vi "Close.vi"(8 "error in (no error)":errorcluster, 11 "PS Driver AMI4xx Actor in":refnum<class "PS Driver AMI4xx.lvclass">) -> (0 "error out":errorcluster, 3 "PS Driver AMI4xx Actor out":refnum<class "PS Driver AMI4xx.lvclass">)   [LabVIEW 2025, in "PS Driver.lvlib" / "PS Driver AMI4xx.lvclass"]
doc: "Author: Scott Hannahs <sth@magnet.fsu.edu>\n\nThis software is licensed for use under the “MIT License\"\nCopyright (c) 2025 Scott Hannahs, sth@sth@magnet.sthnet.net\n\nPermission is hereby granted, free of charge, to any person obtaining a copy of this software and associated documentation files (the \"Software\"), to deal in the Software without restriction, including without limitation the rights to use, copy, modify, merge, publish, distribute, sublicense, and/or sell copies of the Software, and to permit persons to whom the Software is furnished to do so, subject to the following conditions: The above copyright notice and this permission notice shall be included in all copies or substantial portions of the Software.\n\nTHE SOFTWARE IS PROVIDED \"AS IS\", WITHOUT WARRANTY OF ANY KIND, EXPRESS OR IMPLIED, INCLUDING BUT NOT LIMITED TO THE WARRANTIES OF MERCHANTABILITY, FITNESS FOR A PARTICULAR PURPOSE AND NONINFRINGEMENT. IN NO EVENT SHALL THE AUTHORS OR COPYRIGHT HOLDERS BE LIABLE FOR ANY CLAIM, DAMAGES OR OTHER LIABILITY, WHETHER IN AN ACTION OF CONTRACT, TORT OR OTHERWISE, ARISING FROM, OUT OF OR IN CONNECTION WITH THE SOFTWARE OR THE USE OR OTHER DEALINGS IN THE SOFTWARE."
uses:
  PS Driver AMI4xx.lvclass
  PS Driver.lvclass/PS Driver.ctl
  PS Driver with Persistence.lvclass
  PS Driver.lvclass
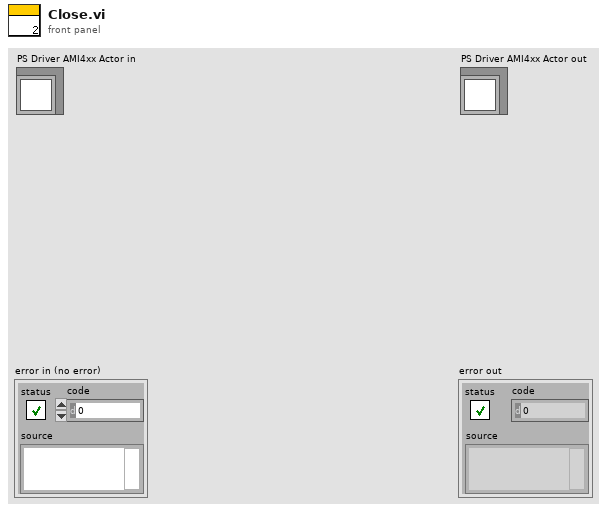
[diagram p1: front panel]
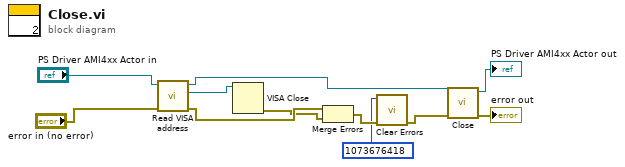
[diagram p0: block diagram]
diagram:
  n1 = call "Read VISA address.vi"("error in (no error)"="error in (no error)", "PS Driver in"="PS Driver AMI4xx Actor in") -> ("error out"=w5:errorcluster, "VISA address"=w9:refnum<visa-resource-name>, "PS Driver out"=w8:refnum<class "PS Driver AMI4xx.lvclass">)  [unwired: 7 in]
  n2 = VISA Close(VISA resource name=w9) -> (error out=w4:errorcluster)  [unwired: 1 in]
  n3 = Merge Errors(w5, w4) -> (w3:errorcluster)
  n4 = call <vilib>:"Clear Errors.vi"("error in (no error)"=w3, "specific error code to clear (0: all)"=1073676418) -> ("error out"=w1:errorcluster)  [unwired: 4 in, 1 out]
  n5 = call-parent "Close.vi"("error in (no error)"=w1, "PS Driver Actor in"=w8) -> ("error out"=→"error out":errorcluster, "PS Driver Actor out"=→"PS Driver AMI4xx Actor out":refnum<class "PS Driver AMI4xx.lvclass">)  [unwired: 8 in]
